vi "gantry_update_speed.vi"(8 "VISA resource name":refnum<visa-resource-name>, 11 "inc/dec":bool) -> (0 "VISA resource name out":refnum<visa-resource-name>, 3 "read buffer":string)   [LabVIEW 2021]
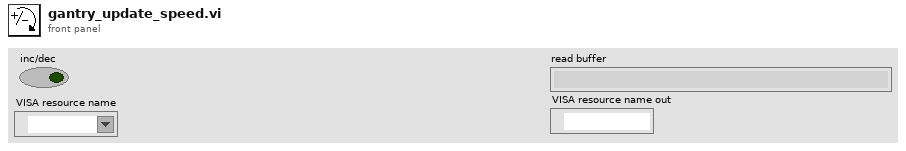
[diagram p1: front panel]
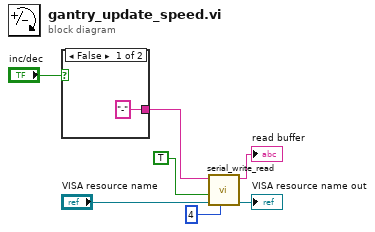
[diagram p0: block diagram]
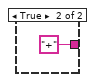
[diagram p2: hidden frame]
diagram:
  n1 = case shown="False" "inc/dec" {
    tunnel: ["-" ("write buffer") "+" ("write buffer")] -> w6
    frame False {
    }
    frame True {
    }
  }
  n2 = call "serial_write_read.vi"("read byte count"=u32 4 ("byte count"), "VISA resource name"="VISA resource name", "Clear buffer"=TRUE, "write buffer"=w6) -> ("VISA resource name out"=→"VISA resource name out":refnum<visa-resource-name>, "read buffer"=→"read buffer":string)  [unwired: 6 in]
